vi "Main.vi"(10 "Acquisition Panel":refnum<vi>, 11 "Module Admin":refnum<class "Delacor_lib_QMH_Module Admin.lvclass">) -> ()   [LabVIEW 2020, in "Acquisition whit helper loop.lvlib"]
doc: "This template is based off of the Queued Message Handler design pattern and the Queued Message Handler project template that ships with LabVIEW.\n\nThe main difference is that the queue is private to this module and communication between modules is performed via Broadcast and Request events.\n\nRequest events are wrapped in public API methods and are handled in the Event Handling Loop (EHL) of this VI. Any module can register for Broadcast events sent by this module. The EHL generates messages based on user interface actions.\n\nThe Message Handling Loop (MHL) processes messages generated by the EHL, or by other messages. The messages are string values, so new messages can be added easily to the Message Cases case structure in the MHL. Each message cluster can also provide an optional value for Message Data, which is a variant that can be converted to whatever message-specific data is required.\n_____\nBased on Delacor QMH Project Template 5.0.0.82."
uses:
  Acquisition whit helper loop.lvlib
  <vilib>/Delacor/Delacor QMH/Libraries/Module Admin_class/Delacor_lib_QMH_Module Admin.lvclass
  Module Data--cluster.ctl
  Stop Argument--cluster.ctl
  <vilib>/Delacor/Delacor QMH/Libraries/Message Queue_class/Delacor_lib_QMH_Message Queue.lvclass/Delacor_lib_QMH_Message Queue.ctl
  <vilib>/Delacor/Delacor QMH/Libraries/Module Admin_class/Delacor_lib_QMH_Module Admin.lvclass/Delacor_lib_QMH_Module Admin.ctl
  set Acquisition Config Argument--cluster.ctl
  <vilib>/Utility/miscctls.llb/LVPointTypeDef.ctl
  Start Acquisition Argument--cluster.ctl
  <vilib>/Delacor/Delacor QMH/Libraries/Message Queue_class/Delacor_lib_QMH_Enqueue Message (Single).vi
  <vilib>/Delacor/Delacor QMH/Libraries/Module Admin_class/Delacor_lib_QMH_Get External Launch.vi
  <vilib>/Utility/error.llb/Error Cluster From Error Code.vi
  <vilib>/ErrorRing/Error Ring.xnode
  <vilib>/Delacor/Delacor QMH/Libraries/Message Queue_class/Delacor_lib_QMH_Message Queue.lvclass
  <vilib>/measure/NI_MABase.lvlib
panel:
  out "Waveform Graph":waveform(dbl)(graph)
  out "error out":errorcluster
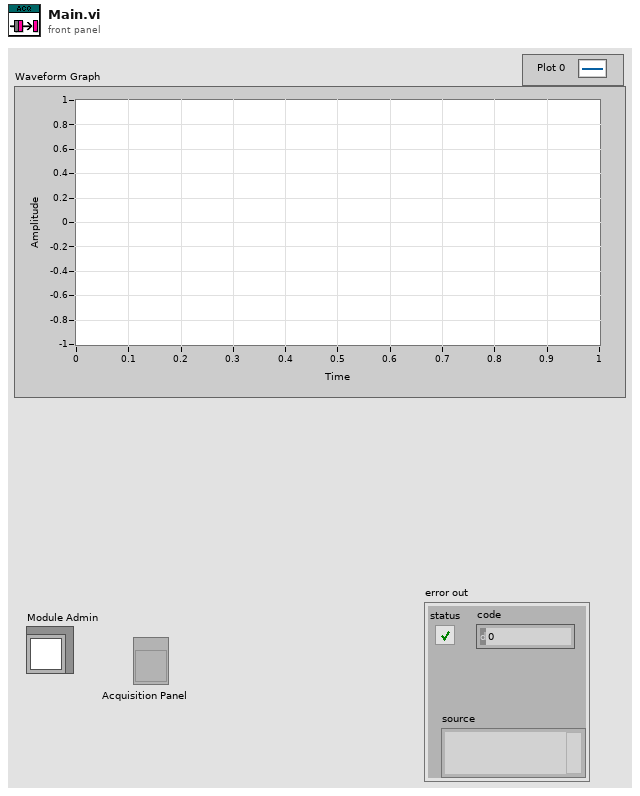
[diagram p1: front panel]
types:
  T1 = typedef "Acquisition whit helper loop.lvlib/Request Events--cluster.ctl" = cluster{"Stop Module":refnum<user-event>, "Show Panel":refnum<user-event>, "Hide Panel":refnum<user-event>, "Get Module Execution Status":refnum<user-event>, "Show Diagram":refnum<user-event>, "Start Helper Loop":refnum<user-event>, "Stop Helper Loop":refnum<user-event>, "set Acquisition Config":refnum<user-event>}
  T2 = typedef "Acquisition whit helper loop.lvlib/Module Data--cluster.ctl" = cluster{"Status":string}
  T3 = enum32{"invalid lock state", "Not Locked", "Locked (No Password)", "Password-protected"}
  T4 = typedef "Acquisition whit helper loop.lvlib/Stop Argument--cluster.ctl" = cluster{"Origin":string, "Exit via Stop Module Req?":bool, "Wait for Module to stop?":bool}
  T5 = typedef "Acquisition whit helper loop.lvlib/set Acquisition Config Argument--cluster.ctl" = cluster{"Config":cluster{"frequency":dbl, "square wave duty cycle (%)":dbl, "phase":dbl, "amplitude":dbl, "signal type":enum16{"Sine Wave", "Triangle Wave", "Square Wave", "Sawtooth Wave"}, "offset":dbl, "sampling info":cluster{"Fs":dbl, "#s":dbl}}}
  T6 = typedef "LVPointTypeDef.ctl" = cluster{"Horizontal":i16, "Vertical":i16}
  T7 = enum32{"Invalid", "Standard", "Closed", "Hidden", "Minimized", "Maximized"}
  T8 = typedef "Start Acquisition Argument--cluster.ctl" = cluster{"Boolean":bool}
  T9 = cluster{"frequency":dbl, "square wave duty cycle (%)":dbl, "phase":dbl, "amplitude":dbl, "signal type":enum16{"Sine Wave", "Triangle Wave", "Square Wave", "Sawtooth Wave"}, "offset":dbl, "sampling info":cluster{"Fs":dbl, "#s":dbl}}
  T10 = enum16{"Sine Wave", "Triangle Wave", "Square Wave", "Sawtooth Wave"}
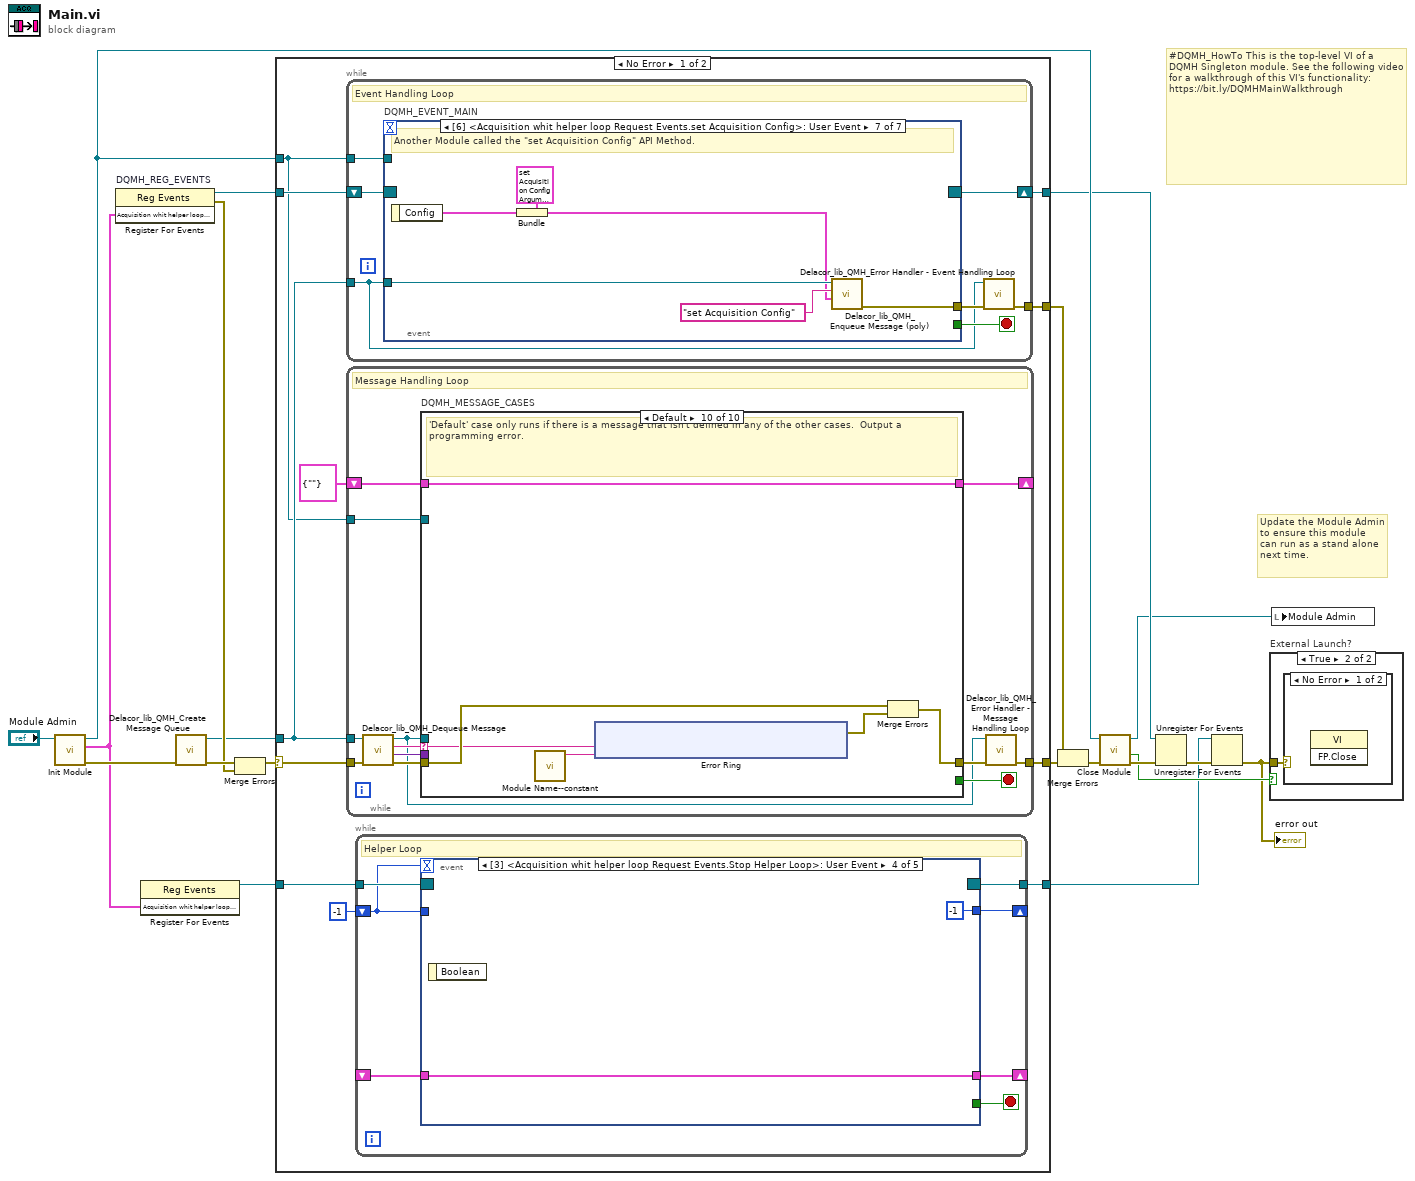
[diagram p0: block diagram]
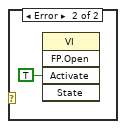
[diagram p3: hidden frame]
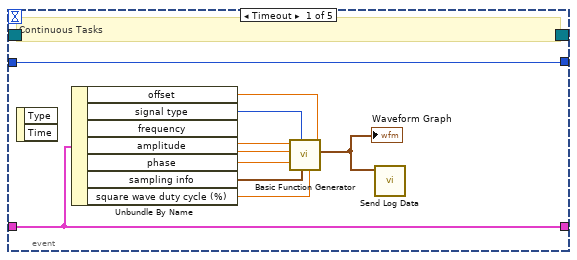
[diagram p4: hidden frame]
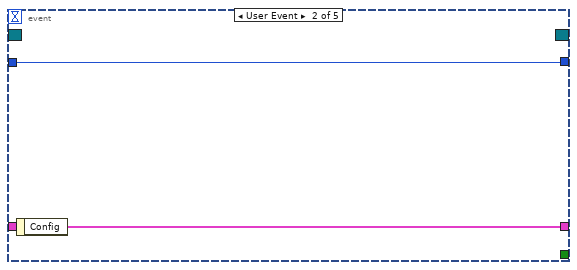
[diagram p5: hidden frame]
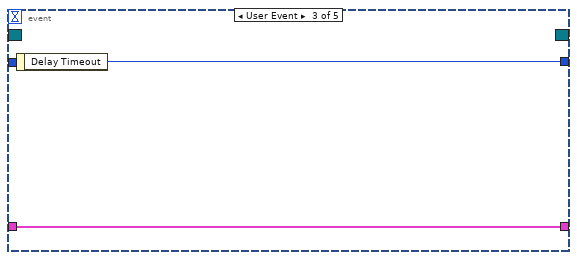
[diagram p6: hidden frame]
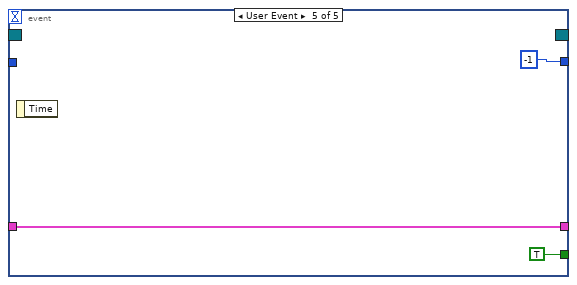
[diagram p7: hidden frame]
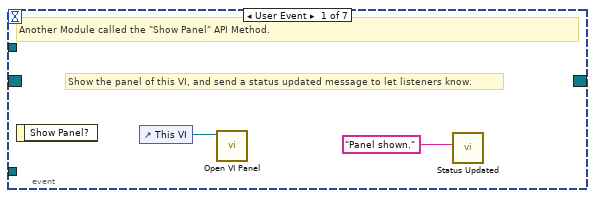
[diagram p8: hidden frame]
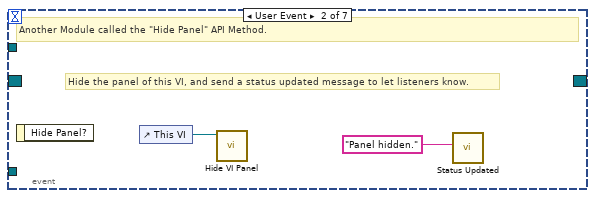
[diagram p9: hidden frame]
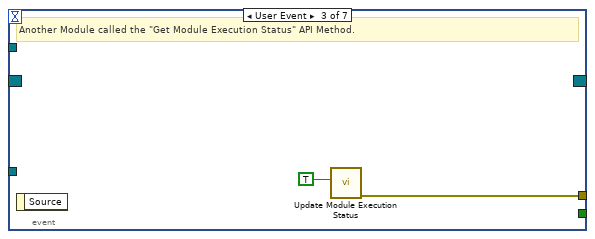
[diagram p10: hidden frame]
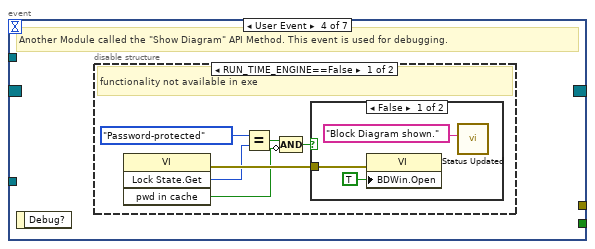
[diagram p11: hidden frame]
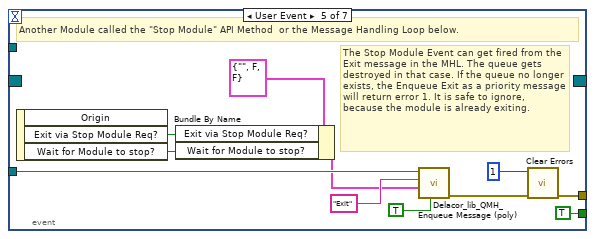
[diagram p14: hidden frame]
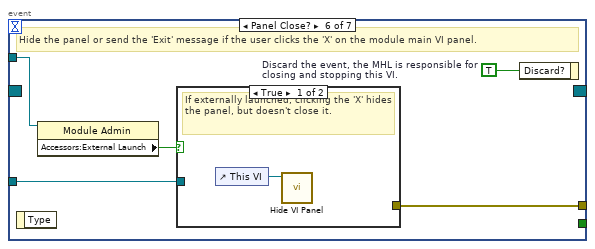
[diagram p15: hidden frame]
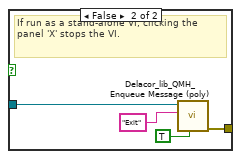
[diagram p16: hidden frame]
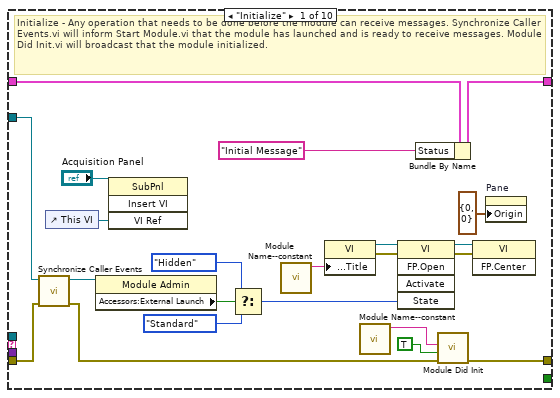
[diagram p17: hidden frame]
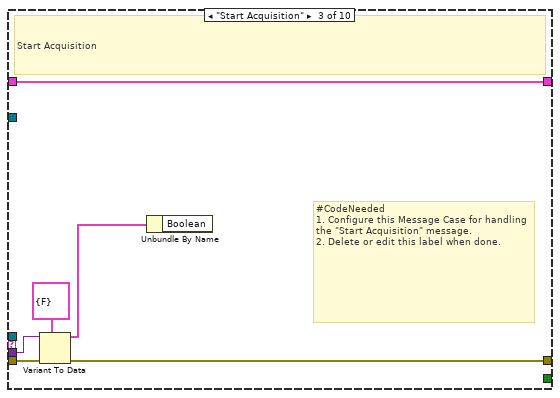
[diagram p19: hidden frame]
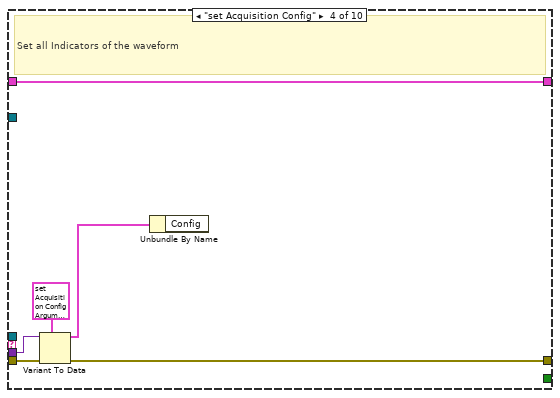
[diagram p20: hidden frame]
diagram:
  # "#DQMH_HowTo This is the top-level VI of a DQMH Singleton module. See the following video for a walkthrough of this VI's functionality: https://bit.ly/DQMHMainWalkthrough"
  # "Update the Module Admin to ensure this module can run as a stand alone next time."
  n1 = call "Init Module.vi"("Singleton Module Admin in"="Module Admin") -> ("error out"=w19:errorcluster, "Acquisition whit helper loop Request Events"=w3:T1, "Singleton Module Admin out"=w11:refnum<class "Delacor_lib_QMH_Module Admin.lvclass">)  [unwired: 8 in]
  n2 = register-events "DQMH_REG_EVENTS"(w3) -> (reference out=w9:refnum<event-registration>, error out=w12:errorcluster)  [unwired: 2 in]
  n3 = register-events(w3) -> (reference out=w4:refnum<event-registration>)  [unwired: 2 in, 1 out]
  n4 = call <vilib>:"Delacor_lib_QMH_Create Message Queue.vi"("error in (no error)"=w19) -> ("error out"=w14:errorcluster, "Message Queue"=w8:refnum<class "Delacor_lib_QMH_Message Queue.lvclass">)  [unwired: 9 in]
  n5 = Merge Errors(w14, w12) -> (w13:errorcluster)
  n6 = case shown="No Error" w13 {
    selector: w13 -> [w29 w221]
    tunnel: [w31 w220] -> w20
    tunnel: [w28 w226] -> w10
    tunnel: w9 -> [w26 w226]
    tunnel: w8 -> [w25 w219]
    tunnel: [w30 _] -> w17
    tunnel: w11 -> [w24 w222]
    tunnel: w4 -> [w23 w218]
    tunnel: [w22 w218] -> w1
    frame No Error {
      n7 = while {
        tunnel: w25 -> [w58]
        shift-right: [w61] -> w28
        shift-left: w26 -> [w62]
        tunnel: [w63] -> w30
        tunnel: w24 -> [w59]
        stop <- w60 stop-if-true
        # "Event Handling Loop"
        n8 = event "DQMH_EVENT_MAIN" shown="[6] <Acquisition whit helper loop Request Events.set Acquisition Config>: User Event" {
          selector: w62 -> [_ _ _ _ _ _ _]
          dyn-events: [_ _ _ _ _ _ _] -> w61
          timeout: _ -> [_ _ _ _ _ _ _]
          tunnel: [_ _ _ _ TRUE ("Discard?") _ _] -> w60
          tunnel: w58 -> [_ _ _ _ w86 w93 w106]
          tunnel: [_ _ w70 _ w89 w95 w101] -> w64
          tunnel: w59 -> [_ _ _ _ _ w92 _]
          event User Event {
            # "Show the panel of this VI, and send a status updated message to let listeners know."
            # "Another Module called the \"Show Panel\" API Method."
            n9 = event-data() -> ()  [unwired: 1 in, 1 out]
            n10 = control-ref of="This VI"() -> (w66:refnum<vi>)
            n11 = call "Open VI Panel.vi"("VI"=w66) -> ()  [unwired: 10 in, 1 out]
            n12 = call "Status Updated.vi"("Status"="Panel shown." ("format string")) -> ()  [unwired: 10 in, 1 out]
          }
          event User Event {
            # "Hide the panel of this VI, and send a status updated message to let listeners know."
            # "Another Module called the \"Hide Panel\" API Method."
            n13 = event-data() -> ()  [unwired: 1 in, 1 out]
            n14 = control-ref of="This VI"() -> (w68:refnum<vi>)
            n15 = call "Hide VI Panel.vi"("VI"=w68) -> ()  [unwired: 10 in, 1 out]
            n16 = call "Status Updated.vi"("Status"="Panel hidden." ("format string")) -> ()  [unwired: 10 in, 1 out]
          }
          event User Event {
            # "Another Module called the \"Get Module Execution Status\" API Method."
            n17 = event-data() -> ()  [unwired: 1 in, 1 out]
            n18 = call "Update Module Execution Status.vi"("Running?"=TRUE) -> ("error out"=w70:errorcluster)  [unwired: 10 in]
          }
          event User Event {
            # "Another Module called the \"Show Diagram\" API Method. This event is used for debugging."
            n19 = event-data() -> ()  [unwired: 1 in, 1 out]
            n20 = disable-structure shown="RUN_TIME_ENGINE==False" {
              frame condition #0 (active) {
                # "functionality not available in exe"
                n21 = invoke class="VI" method="Lock State.Get"() -> (error out=w76:errorcluster, "Get Lock State"=w75:T3, "pwd in cache"=w72:bool)  [unwired: 4 in, 1 out]
                n22 = Equal?(x=T3."Password-protected", y=w75) -> (x = y?=w73:bool)
                n23 = Compound Arithmetic op=AND(w73, invert w72) -> (w71:bool)
                n24 = case shown="False" w71 {
                  tunnel: w76 -> [w79 _]
                  frame False {
                    n25 = property class="VI"(error in=w79, "BDWin.Open"=TRUE ("Block Diagram Window:Open")) -> ()  [unwired: 1 in, 2 out]
                    n26 = call "Status Updated.vi"("Status"="Block Diagram shown." ("format string")) -> ()  [unwired: 10 in, 1 out]
                  }
                  frame True {
                    # "Password-protected VI, and the password is not in the cache. Do not show the diagram."
                  }
                }
              }
              frame condition #1 {
              }
            }
          }
          event User Event {
            # "The Stop Module Event can get fired from the Exit message in the MHL. The queue gets destroyed in that case. If the queue no longer exists, the Enqueue Exit as a priority message will return error 1. It is safe to ignore, because the module is already exiting."
            # "Another Module called the \"Stop Module\" API Method  or the Message Handling Loop below."
            n27 = event-data() -> ("Exit via Stop Module Req?"=w82:bool, "Wait for Module to stop?"=w81:bool)  [unwired: 1 in, 1 out]
            n28 = Bundle By Name(cluster=T4 {"Origin"="", "Exit via Stop Module Req?"=FALSE, "Wait for Module to stop?"=FALSE} ("Stop Argument"), "Exit via Stop Module Req?"=w82, "Wait for Module to stop?"=w81) -> (w80:T4)
            n29 = call-poly <vilib>:"Delacor_lib_QMH_Enqueue Message (poly).vi"("Priority Message? (F)"=TRUE, "Message Data"=w80, "Message"="Exit", "Message Queue in"=w86) -> ("error out"=w90:errorcluster)  [unwired: 6 in, 1 out]
            n30 = call <vilib>:"Clear Errors.vi"("error in (no error)"=w90, "specific error code to clear (0: all)"=1) -> ("error out"=w89:errorcluster)  [unwired: 4 in, 1 out]
          }
          event Panel Close? {
            w94 = TRUE  # Discard the event, the MHL is responsible for closing and stopping this VI.
            # "Hide the panel or send the 'Exit' message if the user clicks the 'X' on the module main VI panel."
            n31 = event-data() -> ()  [unwired: 1 in, 1 out]
            n32 = property class="Module Admin"(reference=w92) -> ("Accessors:External Launch"=w91:bool)  [unwired: 1 in, 2 out]
            n33 = case shown="True" w91 {
              tunnel: w93 -> [_ w99]
              tunnel: [_ w100] -> w95
              frame True {
                # "If externally launched, clicking the 'X' hides the panel, but doesn't close it."
                n34 = control-ref of="This VI"() -> (w96:refnum<vi>)
                n35 = call "Hide VI Panel.vi"("VI"=w96) -> ()  [unwired: 10 in, 1 out]
              }
              frame False {
                # "If run as a stand-alone VI, clicking the panel 'X' stops the VI."
                n36 = call-poly <vilib>:"Delacor_lib_QMH_Enqueue Message (poly).vi"("Priority Message? (F)"=TRUE, "Message"="Exit", "Message Queue in"=w99) -> ("error out"=w100:errorcluster)  [unwired: 7 in, 1 out]
              }
            }
            n37 = event-data("Discard?"=w94) -> ()  [unwired: 1 in, 1 out]
          }
          event User Event {
            # "Another Module called the \"set Acquisition Config\" API Method."
            n38 = event-data() -> ("Config"=w102:T9)  [unwired: 1 in]
            n39 = Bundle(cluster=T5 {"Config"={"frequency"=10.0, "square wave duty cycle (%)"=50.0, "phase"=0.0, "amplitude"=1.0, "signal type"=enum."Sine Wave", "offset"=0.0, "sampling info"={"Fs"=1000.0, "#s"=1000.0}}} ("set Acquisition Config Argument"), "Config"=w102) -> (w103:T5)
            n40 = call-poly <vilib>:"Delacor_lib_QMH_Enqueue Message (poly).vi"("Message Data"=w103, "Message"="set Acquisition Config", "Message Queue in"=w106) -> ("error out"=w101:errorcluster)  [unwired: 7 in, 1 out]
          }
        }
        n41 = call-dynamic "Delacor_lib_QMH_Error Handler - Event Handling Loop.vi"("error in (no error)"=w64, "Message Queue in"=w58) -> ("dup error in"=w63:errorcluster)  [unwired: 8 in, 1 out]
      }
      n42 = while {
        tunnel: w25 -> [w109]
        shift-right: [w113] -> _
        shift-left: T2 {"Status"=""} ("Data Cluster") -> [w114]
        tunnel: w29 -> [w117]
        tunnel: [w115] -> w31
        tunnel: w24 -> [w107]
        stop <- w112 stop-if-true
        # "Message Handling Loop"
        n43 = call-dynamic "Delacor_lib_QMH_Dequeue Message.vi"("error in (no error)"=w117, "Message Queue in"=w109) -> ("error out"=w116:errorcluster, "Message Data"=w110:variant, "Message"=w111:string, "Message Queue out"=w108:refnum<class "Delacor_lib_QMH_Message Queue.lvclass">)  [unwired: 6 in]
        n44 = case "DQMH_MESSAGE_CASES" shown="Default" w111 {
          selector: w111 -> [_ _ _ _ _ _ _ _ _ w205]
          tunnel: w108 -> [_ _ _ _ _ _ _ w175 w197 _]
          tunnel: w116 -> [w138 w142 w148 w154 w157 w159 w164 w182 w203 w207]
          tunnel: [w136 w142 w146 w152 w156 w159 w163 w178 w200 w208] -> w118
          tunnel: w114 -> [w127 w141 w147 w153 w155 w158 w161 w177 w196 w206]
          tunnel: [w126 w141 w147 w153 w155 w158 w161 w177 w196 w206] -> w113
          tunnel: [_ _ _ _ _ _ _ _ w195 _] -> w112
          tunnel: w110 -> [_ _ w145 w151 _ _ _ w176 w194 _]
          tunnel: w107 -> [w128 _ _ _ _ _ _ w174 w189 _]
          frame "Initialize" {
            # "Initialize - Any operation that needs to be done before the module can receive messages. Synchronize Caller Events.vi will inform Start Module.vi that the module has launched and is ready to receive messages. Module Did Init.vi will broadcast that the module initialized."
            n45 = call "Synchronize Caller Events.vi"("error in (no error)"=w138, "Singleton Module Admin in"=w128) -> ("error out"=w137:errorcluster, "Singleton Module Admin out"=w123:refnum<class "Delacor_lib_QMH_Module Admin.lvclass">)  [unwired: 8 in]
            n46 = control-ref of="This VI"() -> (w119:refnum<vi>)
            n47 = property class="Module Admin"(reference=w123) -> ("Accessors:External Launch"=w132:bool)  [unwired: 1 in, 2 out]
            n48 = invoke class="SubPnl" method="Insert VI"(reference="Acquisition Panel", "VI Ref"=w119) -> ()  [unwired: 2 in, 4 out]
            n49 = Select(t=T7."Hidden" ("State"), s=w132, f=T7."Standard" ("State")) -> (s? t:f=w129:T7)
            n50 = call "Module Name--constant.vi"() -> ("Module Name"=w135:string)  [unwired: 11 in]
            n51 = property class="VI"("Front Panel.Title"=w135) -> (reference out=w134:refnum<vi>, error out=w140:errorcluster)  [unwired: 2 in]
            n52 = call "Module Name--constant.vi"() -> ("Module Name"=w124:string)  [unwired: 11 in]
            n53 = invoke class="VI" method="FP.Open"(reference=w134, error in=w140, "State"=w129) -> (reference out=w133:refnum<vi>, error out=w139:errorcluster)  [unwired: 2 in, 3 out]
            n54 = Bundle By Name(cluster=w127, "Status"="Initial Message" ("Initial Message")) -> (w126:T2)
            n55 = call "Module Did Init.vi"("error in (no error)"=w137, "Initialized?"=TRUE, "Origin"=w124) -> ("error out"=w136:errorcluster)  [unwired: 8 in]
            n56 = invoke class="VI" method="FP.Center"(reference=w133, error in=w139) -> ()  [unwired: 1 in, 3 out]
            n57 = property on="Pane" class="Pane"("Origin"=T6 {"Horizontal"=0, "Vertical"=0}) -> ()  [unwired: 2 in, 2 out]
          }
          frame "--- Module Specific ---" {
            # "Separator -- The following cases handle messages specific to this Module."
          }
          frame "Start Acquisition" {
            # "#CodeNeeded\n1. Configure this Message Case for handling the \"Start Acquisition\" message.\n2. Delete or edit this label when done."
            # "Start Acquisition"
            n58 = Variant To Data(error in=w148, type=T8 {"Boolean"=FALSE} ("Start Acquisition Argument"), Variant=w145) -> (data=w143:T8, error out=w146:errorcluster)
            n59 = Unbundle By Name(w143) -> ()  [unwired: 1 out]
          }
          frame "set Acquisition Config" {
            # "Set all Indicators of the waveform"
            n60 = Variant To Data(error in=w154, type=T5 {"Config"={"frequency"=10.0, "square wave duty cycle (%)"=50.0, "phase"=0.0, "amplitude"=1.0, "signal type"=enum."Sine Wave", "offset"=0.0, "sampling info"={"Fs"=1000.0, "#s"=1000.0}}} ("set Acquisition Config Argument"), Variant=w151) -> (data=w149:T5, error out=w152:errorcluster)
            n61 = Unbundle By Name(w149) -> ()  [unwired: 1 out]
          }
          frame "---Copy This Frame---" {
            # "Duplicate this frame when creating new messages.  Change this comment in the duplicated frame to describe this message."
            n62 = Merge Errors(w157) -> (w156:errorcluster)
          }
          frame "--- Exit and Error Handling---" {
            # "Separator - The following cases handle errors and exit messages."
          }
          frame "Simulate MHL Error" {
            # "#DQMH_HowTo The 'Simulate MHL Error' button  illustrates how the MHL handles errors. This event is instructional in nature and can be removed."
            # "Simulate an error occurring at the MHL"
            n63 = call "Module Name--constant.vi"() -> ("Module Name"=w160:string)  [unwired: 11 in]
            n64 = xnode "Error Ring"("parameter 0"=w160) -> ("error out"=w162:errorcluster)
            n65 = Merge Errors(w164, w162) -> (w163:errorcluster)
          }
          frame "Error" {
            # "#CodeRecommended - If you ever change the name of this \"Error\" message, you'll need to update the name in the Check Loop Error.vi as well."
            # "#CodeRecommended - If the module is running in standalone mode (External Launch = FALSE), this code will pop up an error dialog and call the 'Exit' message if an error occurs. Add more fine-grained error handling here."
            # "Error - Check the error message data and respond accordingly. This message is sent by the \"Error Handler\" VIs at the end of each loop in this application."
            n66 = property class="Module Admin"(reference=w174) -> ("Accessors:External Launch"=w173:bool)  [unwired: 1 in, 2 out]
            n67 = Variant To Data(error in=w182, type=errorcluster {"status"=FALSE, "code"=0, "source"=""} ("error constant"), Variant=w176) -> (data=w183:errorcluster, error out=w180:errorcluster)
            n68 = call "Module Name--constant.vi"() -> ("Module Name"=w172:string)  [unwired: 11 in]
            n69 = call "Error Reported.vi"("Additional Information"=w172, "Error"=w183) -> ()  [unwired: 9 in, 1 out]
            n70 = case shown="False" w173 {
              tunnel: [w188 _] -> w179
              tunnel: w175 -> [w186 _]
              tunnel: w183 -> [w187 _]
              frame False {
                # "If the module is running standalone, then pop up an error dialog and call the \"Exit\" message."
                n71 = call <vilib>:"Simple Error Handler.vi"("error in (no error)"=w187) -> ()  [unwired: 4 in, 5 out]
                n72 = call-poly <vilib>:"Delacor_lib_QMH_Enqueue Message (poly).vi"("Priority Message? (F)"=TRUE, "Message"="Exit", "Message Queue in"=w186) -> ("error out"=w188:errorcluster)  [unwired: 7 in, 1 out]
              }
              frame True {
                # "If the module was launched externally, calling the Error Reported broadcast VI is the only action performed by the \"Error\" message. The module's caller can then process the error appropriately."
              }
            }
            n73 = Merge Errors(w180, w179) -> (w178:errorcluster)
            n74 = local write "error out"(w178) -> ()
          }
          frame "Exit" {
            w193 = 91  # 91: not all Exit messages will have an argument
            w195 = TRUE  # Stop the VI
            # "Release the message queue reference"
            # "#CodeNeeded - Add any required cleanup code here"
            # "Exit - Exit the application."
            n75 = Variant To Data(error in=w203, type=T4 {"Origin"="", "Exit via Stop Module Req?"=FALSE, "Wait for Module to stop?"=FALSE} ("Stop Argument"), Variant=w194) -> (data=w191:T4, error out=w199:errorcluster)
            n76 = call <vilib>:"Clear Errors.vi"("error in (no error)"=w199, "specific error code to clear (0: all)"=w193) -> ("error out"=w202:errorcluster)  [unwired: 4 in, 1 out]
            n77 = control-ref of="This VI"() -> (w190:refnum<vi>)
            n78 = call-dynamic "Delacor_lib_QMH_Release Message Queue.vi"("error in (no error)"=w202, "Message Queue"=w197) -> ("error out"=w201:errorcluster)  [unwired: 9 in]
            n79 = call "Handle Exit.vi"("Stop Argument"=w191, "Admin in"=w189, "VI reference"=w190) -> ("error out"=w198:errorcluster)  [unwired: 7 in, 1 out]
            n80 = Merge Errors(w201, w198) -> (w200:errorcluster)
          }
          frame Default {
            # "'Default' case only runs if there is a message that isn't defined in any of the other cases.  Output a programming error."
            n81 = call "Module Name--constant.vi"() -> ("Module Name"=w204:string)  [unwired: 11 in]
            n82 = xnode "Error Ring"("parameter 0"=w205, "parameter 1"=w204) -> ("error out"=w209:errorcluster)
            n83 = Merge Errors(w207, w209) -> (w208:errorcluster)
          }
        }
        n84 = call-dynamic "Delacor_lib_QMH_Error Handler - Message Handling Loop.vi"("error in (no error)"=w118, "Message Queue in"=w108) -> ("dup error in"=w115:errorcluster)  [unwired: 8 in, 1 out]
      }
      n85 = while {
        tunnel: w23 -> [w38]
        tunnel: [w37] -> w22
        shift-right: [w36] -> _
        shift-left: -1 -> [w35]
        shift-right: [w33] -> _
        shift-left: _ -> [w32]
        stop <- w34 stop-if-true
        # "Helper Loop"
        n86 = event shown="[3] <Acquisition whit helper loop Request Events.Stop Helper Loop>: User Event" {
          selector: w38 -> [_ _ _ _ _]
          dyn-events: [_ _ _ _ _] -> w37
          timeout: w35 -> [_ _ _ _ _]
          tunnel: [w48 w49 w52 -1 -1] -> w36
          tunnel: w35 -> [w48 w49 _ _ _]
          tunnel: [_ _ _ _ TRUE] -> w34
          tunnel: [w47 w50 w51 w53 w55] -> w33
          tunnel: w32 -> [w47 _ w51 w53 w55]
          event Timeout {
            # "Continuous Tasks"
            n87 = event-data() -> ()  [unwired: 1 in, 2 out]
            n88 = Unbundle By Name(w47) -> ("offset"=w40:dbl, "signal type"=w46:T10, "frequency"=w45:dbl, "amplitude"=w44:dbl, "phase"=w43:dbl, "sampling info"=w42:cluster{"Fs":dbl, "#s":dbl}, "square wave duty cycle (%)"=w41:dbl)
            n89 = call <vilib>:"Basic Function Generator.vi"("offset"=w40, "square wave duty cycle (%)"=w41, "sampling info"=w42, "signal type"=w46, "phase"=w43, "amplitude"=w44, "frequency"=w45) -> ("signal out"=w39:waveform(dbl))  [unwired: 2 in, 2 out]
            "Waveform Graph" <- w39
            n90 = call "Send Log Data.vi"("signal in"=w39) -> ()  [unwired: 11 in]
          }
          event User Event {
            n91 = event-data() -> ("Config"=w50:T9)  [unwired: 1 in]
          }
          event User Event {
            n92 = event-data() -> ("Delay Timeout"=w52:i32)  [unwired: 1 in]
          }
          event User Event {
            n93 = event-data() -> ()  [unwired: 1 in, 1 out]
          }
          event User Event {
            n94 = event-data() -> ()  [unwired: 1 in, 1 out]
          }
        }
      }
    }
    frame Error {
      # "Synchronize Caller Events.vi will inform Start Module.vi that the module has launched and will let the code calling Start Module.vi register for broadcasts and would permit the caller receive the broadcast that an error occurred at launch time."
      n95 = call-dynamic "Delacor_lib_QMH_Release Message Queue.vi"("error in (no error)"=w221, "Message Queue"=w219) -> ("error out"=w220:errorcluster)  [unwired: 9 in]
      n96 = call "Synchronize Caller Events.vi"("Singleton Module Admin in"=w222) -> ("error out"=w227:errorcluster)  [unwired: 9 in, 1 out]
      n97 = call "Module Name--constant.vi"() -> ("Module Name"=w225:string)  [unwired: 11 in]
      n98 = Format Into String(format string="An error occurred during initialization. %s is no longer running.", w225) -> (resulting string=w223:string)  [unwired: 2 in, 1 out]
      n99 = Merge Errors(w220, w227) -> (w228:errorcluster)
      n100 = call "Error Reported.vi"("Additional Information"=w223, "Error"=w228) -> ()  [unwired: 9 in, 1 out]
    }
  }
  n101 = Merge Errors(w17, w20) -> (w16:errorcluster)
  n102 = call "Close Module.vi"("error in (no error)"=w16, "Module Admin in"=w11) -> ("error out"=w18:errorcluster, "External Launch"=w5:bool, "Module Admin out"=w6:refnum<class "Delacor_lib_QMH_Module Admin.lvclass">)  [unwired: 7 in]
  n103 = Unregister For Events(event registration refnum=w10, error in=w18) -> (error out=w15:errorcluster)
  n104 = Unregister For Events(event registration refnum=w1, error in=w15) -> (error out=w2:errorcluster)
  "error out" <- w2
  n105 = case "External Launch?" shown="True" w5 {
    tunnel: w2 -> [_ w229]
    frame False {
    }
    frame True {
      n106 = case shown="No Error" w229 {
        frame No Error {
          n107 = invoke class="VI" method="FP.Close"() -> ()  [unwired: 3 in, 3 out]
        }
        frame Error {
          n108 = invoke class="VI" method="FP.Open"("Activate"=TRUE ("Activate?")) -> ()  [unwired: 4 in, 5 out]
        }
      }
    }
  }
  n109 = local write "Module Admin"(w6) -> ()
